vi "String to 1D array.vi"(0 "Readed paths":string, 11 "error in":errorcluster) -> (4 "string array":string[](array[string]), 8 "Array size":i32, 15 "error out":errorcluster)   [LabVIEW 2020, in "Custom Sort Function.lvlib"]
doc: "This Vi is used to convert the string to 1D array of strings"
uses:
  Custom Sort Function.lvlib
panel:
  out "source out":string
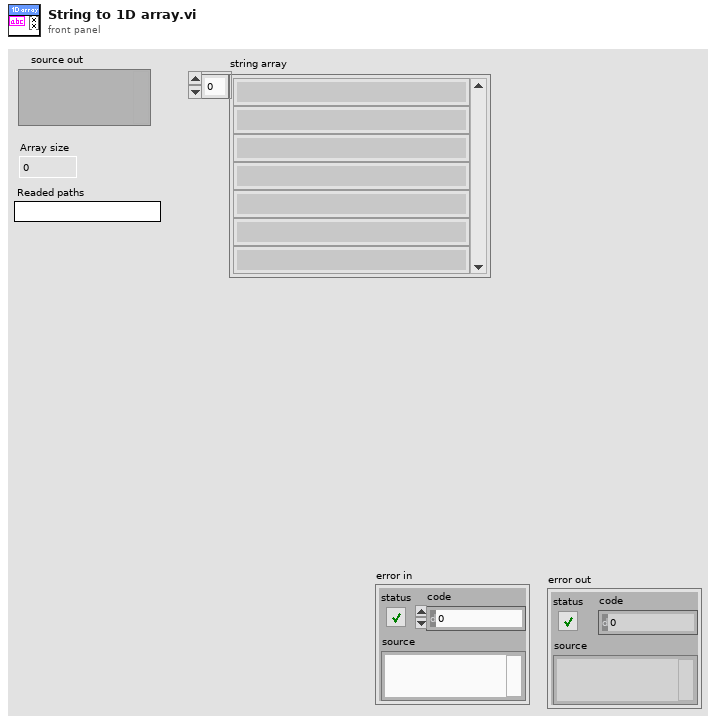
[diagram p1: front panel]
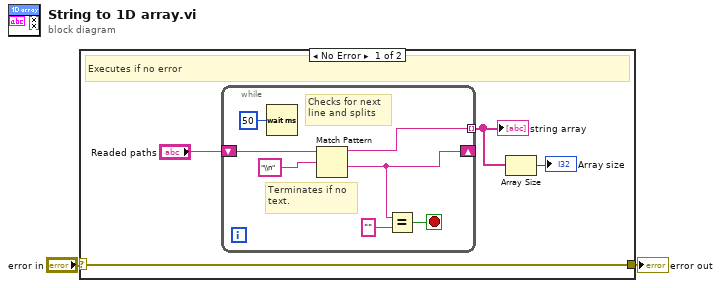
[diagram p0: block diagram]
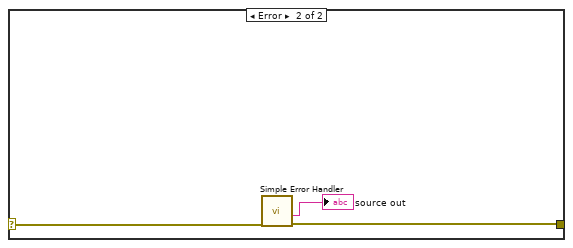
[diagram p2: hidden frame]
diagram:
  n1 = case shown="No Error" "error in" {
    selector: "error in" -> [w4 w16]
    tunnel: [w4 w15] -> w2
    frame No Error {
      # "Executes if no error"
      n2 = while {
        shift-right: [w10] -> _
        shift-left: "Readed paths" -> [w12]
        tunnel: [w7] -> w6 mode=indexing
        stop <- w8 stop-if-true
        # "Checks for next\nline and splits"
        # "Terminates if no \ntext."
        n3 = Wait (ms)(milliseconds to wait=u32 50) -> ()  [unwired: 1 out]
        n4 = Match Pattern(string=w12, regular expression="\\n") -> (before substring=w7:string, after substring=w10:string)  [unwired: 1 in, 2 out]
        n5 = Equal?(x=w10, y="") -> (x = y?=w8:bool)
      }
      "string array" <- w6
      n6 = Array Size(array=w6) -> (size(s)=→"Array size":i32)
    }
    frame Error {
      n7 = call <vilib>:"Simple Error Handler.vi"("error in (no error)"=w16) -> ("source out"=→"source out":string, "error out"=w15:errorcluster)  [unwired: 4 in, 3 out]
    }
  }
  "error out" <- w2
